vi "Out_S7F2.vi"(8 "error in (no error)":errorcluster, 10 "S7F2":T1, 11 "S7 Message Class in":refnum<class "S7 Message Class.lvclass">) -> (0 "error out":errorcluster, 3 "S7 Message Class out":refnum<class "S7 Message Class.lvclass">)   [LabVIEW 2020, in "SECS Communication.lvlib" / "S7 Message Class.lvclass"]
uses:
  S7 Message Class.lvclass
  D:/Dropbox/SECS/LabVIEW Code/Com/SECS Communication/SECS-II Class/SECS-II Class.lvclass
  S7F2.ctl
  SECS-II Class/Data Message_Binary.vi
  S7 Message Class.lvclass/S7 Message Class.ctl
  SECS-II Class/SECS-II Class.lvclass
  D:/Dropbox/SECS/LabVIEW Code/Com/SECS Communication/S7 Message Class/S7 Message Class.lvclass
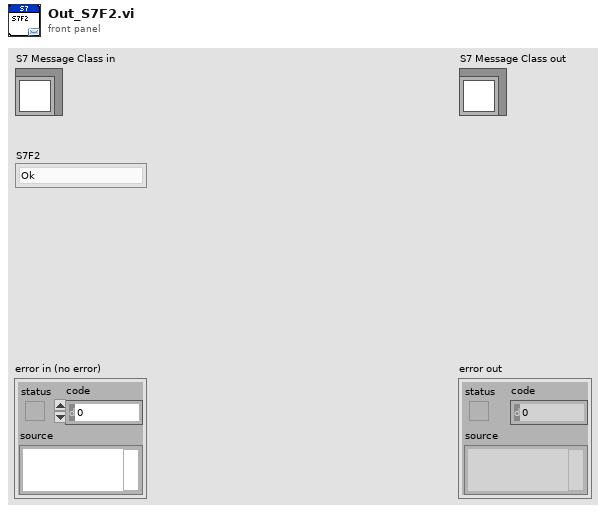
[diagram p1: front panel]
types:
  T1 = typedef "SECS Communication.lvlib/S7 Message Class.lvclass/S7F2.ctl" = enum8{"Ok", "already have", "no space", "invalid PPID", "busy, try later", "will not accept", " other error"}
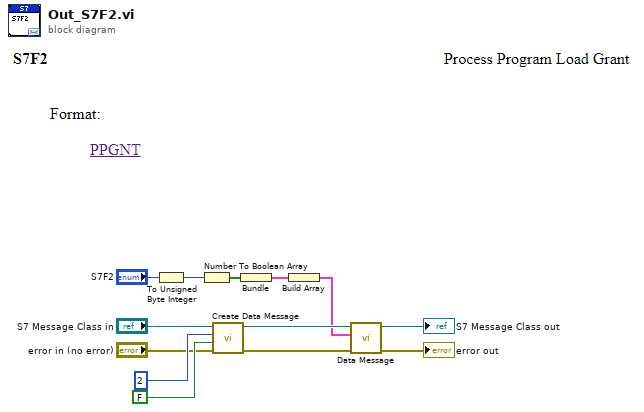
[diagram p0: block diagram]
diagram:
  n1 = To Unsigned Byte Integer(number="S7F2") -> (unsigned 8bit integer=w9:u8)
  n2 = Number To Boolean Array(number=w9) -> (Boolean array=w8:bool[])
  n3 = call "Create Data Message.vi"("error in (no error)"="error in (no error)", "W-Bit"=FALSE, "Function"=u8 2, "SECS-II Class in"="S7 Message Class in") -> ("error out"=w4:errorcluster, "SECS-II Class out"=w6:refnum<class "S7 Message Class.lvclass">)  [unwired: 6 in]
  n4 = Bundle("Boolean array"=w8) -> (w7:cluster{"Boolean array":bool[]})  [unwired: 1 in]
  n5 = Build Array(w7) -> (w1:cluster{"Boolean array":bool[]}[])
  n6 = call-poly "Data Message.vi"("error in"=w4, "Data Cluster"=w1, "SECS-II Class in"=w6) -> ("error out"=→"error out":errorcluster, "SECS-II Class out"=→"S7 Message Class out":refnum<class "S7 Message Class.lvclass">)  [unwired: 7 in]
